vi "Clear HWI.vi"(8 "error in (no error)":errorcluster, 11 "NI Card in":refnum<class "NI Card.lvclass">) -> (0 "error out":errorcluster, 3 "NI Card out":refnum<class "NI Card.lvclass">)   [LabVIEW 2013, in "NI Card.lvclass"]
uses:
  NI Card.lvclass
  NI Card.lvclass/NI Card.ctl
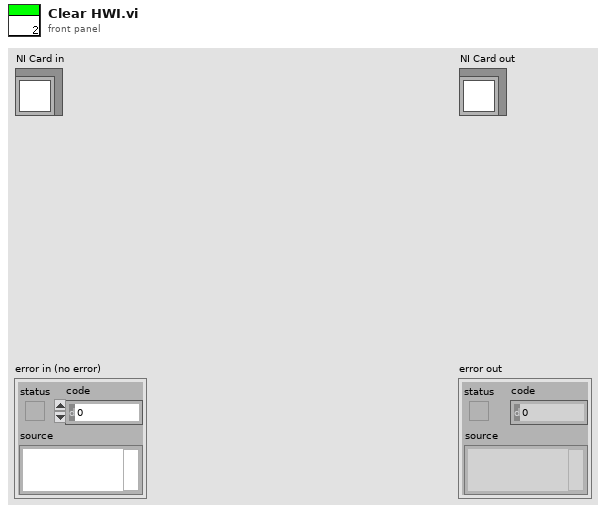
[diagram p1: front panel]
types:
  T1 = cluster{"Analog Output ":dbl[][], "Digital Output":bool[][], "AI Task Out":refnum<k21>, "AO Tasks Out":refnum<k21>[]}
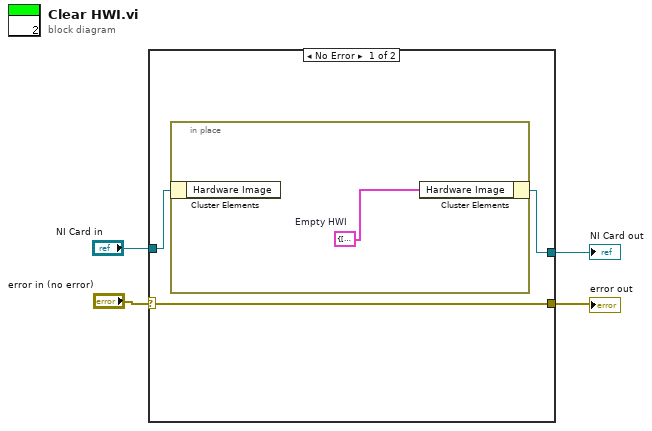
[diagram p0: block diagram]
diagram:
  n1 = case shown="No Error" "error in (no error)" {
    selector: "error in (no error)" -> [w7 w10]
    tunnel: [w7 w10] -> w3
    tunnel: [w5 w9] -> w2
    tunnel: "NI Card in" -> [w6 w9]
    frame No Error {
      n2 = in-place {
        w8 = T1 {"Analog Output "=[], "Digital Output"=[], "AI Task Out"="", "AO Tasks Out"=[]}  # Empty HWI
        n3 = in-place-cluster #1(w6) -> ()  [unwired: 1 out]
        n4 = in-place-cluster #1("Hardware Image"=w8) -> (w5:refnum<class "NI Card.lvclass">)
      }
    }
    frame Error {
    }
  }
  "error out" <- w3
  "NI Card out" <- w2
